vi "Motors sequence 2.vi"(0 "LINX Resource":T1, 1 "Current State":refnum<vi>, 3 "Pole move(microS)":u16(slide) scale=1000.0..2000.0, 4 "Speed(Steps/s)":u32, 5 "Error In":errorcluster, 7 "Wheel":bool, 8 "Spin time/Rest(1)":u32, 9 "Spin n loops":u32=1, 12 "Spin time(2)":u32, 13 "Speed(Steps/s) 2":u32, 14 "Direction":enum16{"CLW", "CCLW", "Off"}(ring), 16 "Pole ms to wait off":u32, 19 "Direction 2":enum16{"CLW", "CCLW", "Off"}(ring), 21 "Seq. iteration 2":refnum<vi>, 22 "Stop":refnum<vi>, 23 "Speed plot 2":refnum<vi>, 24 "Seq. loop":i32, 26 "Spin iteration 2":refnum<vi>) -> (25 "Seq. iteration":i32, 27 "error out":errorcluster)   [LabVIEW 2020]
uses:
  <vilib>/MakerHub/LINX/Private/Type Defs/LINX Ref.ctl
  <vilib>/MakerHub/LINX/Private/Type Defs/Platform.ctl
  <vilib>/MakerHub/LINX/Private/Type Defs/Interface.ctl
  <vilib>/MakerHub/LINX/Private/Device/Type Defs/LINX Device Config.ctl
  <vilib>/MakerHub/LINX/Private/Device/Type Defs/TCP Config.ctl
  <vilib>/MakerHub/LINX/Private/Device/Type Defs/Channels.ctl
  <vilib>/MakerHub/LINX/Public/Sensors/Motion/Servo/Servo Set Pulse Width One Channel.vi
  <vilib>/MakerHub/LINX/Public/Sensors/Motion/Servo/Servo.lvlib
  <vilib>/MakerHub/LINX/LMH-LINX.lvlib
  <vilib>/MakerHub/LINX/Private/Device/Device.lvlib
panel:
  out "Suggested P2 time":u32
  out "Speed plot":dbl(graph)
  out "Spin iteration":i32
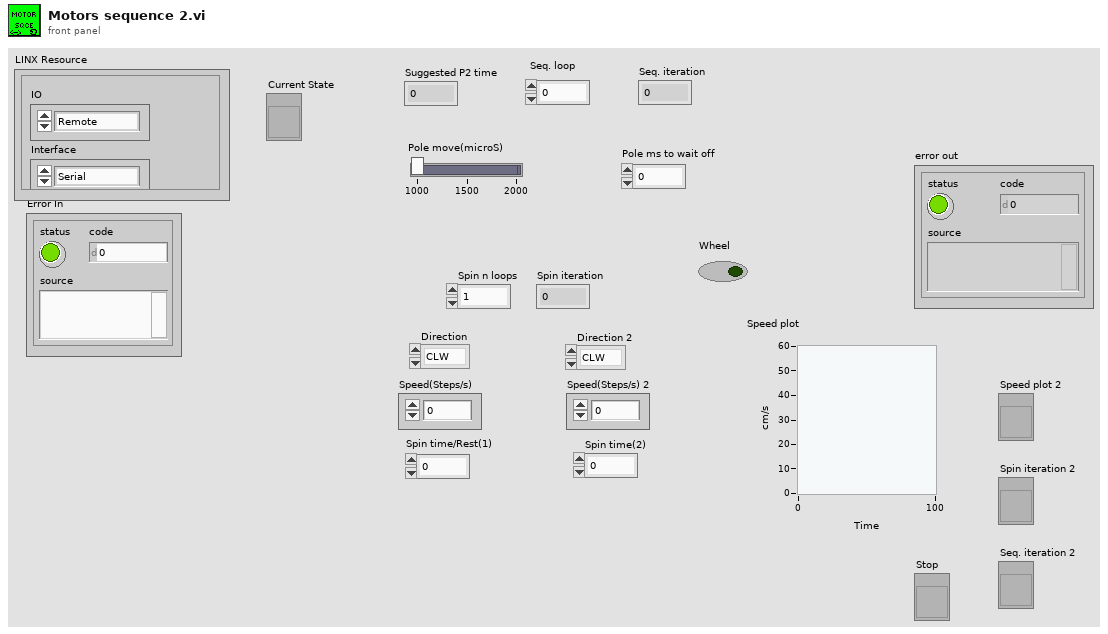
[diagram p1: front panel]
types:
  T1 = typedef "LMH-LINX.lvlib/LINX Ref.ctl" = cluster{"IO":T2, "Interface":T3, "LINX Device Config":T4}
  T2 = typedef "LMH-LINX.lvlib/Platform.ctl" = enum16{"Remote", "Local"}
  T3 = typedef "LMH-LINX.lvlib/Interface.ctl" = enum16{"Serial", "TCP"}
  T4 = typedef "LMH-LINX.lvlib/Device.lvlib/LINX Device Config.ctl" = cluster{"Interface":T3, "COM Port":refnum<visa-resource-name>, "TCP Configuration":T5, "Device Family":u8, "Device ID":u8, "Device Name":string, "TCP Ref":refnum<k5>, "Channels":T6}
  T5 = typedef "LMH-LINX.lvlib/Device.lvlib/TCP Config.ctl" = cluster{"IP Address":string, "Port":u16}
  T6 = typedef "LMH-LINX.lvlib/Channels.ctl" = cluster{"DI":u8[], "DO":u8[], "AI":u8[], "AO":u8[], "PWM":u8[], "QE":u8[], "UART":u8[], "I2C 2":u8[], "SPI":u8[], "CAN":u8[], "Servo":u8[], "AI Ref (V)":dbl, "AI Resolution (Bits)":u8, "AO Ref (V)":dbl, "AO Resolution (Bits)":u8}
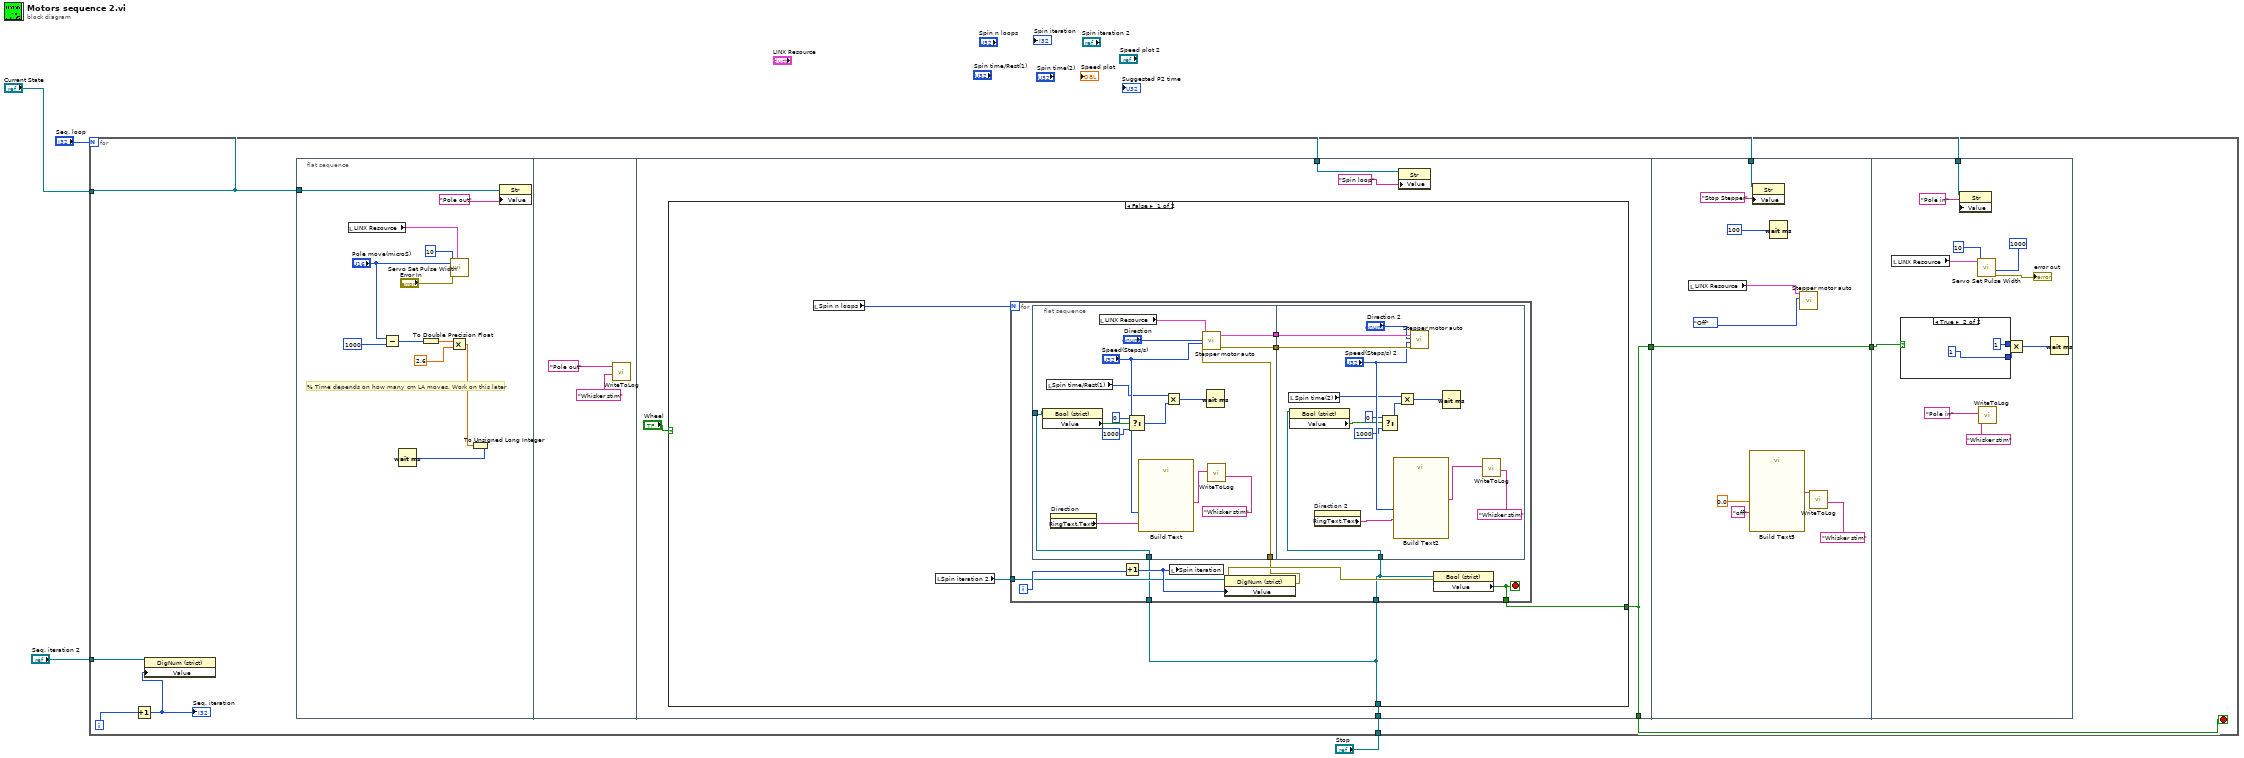
[diagram p0: block diagram]
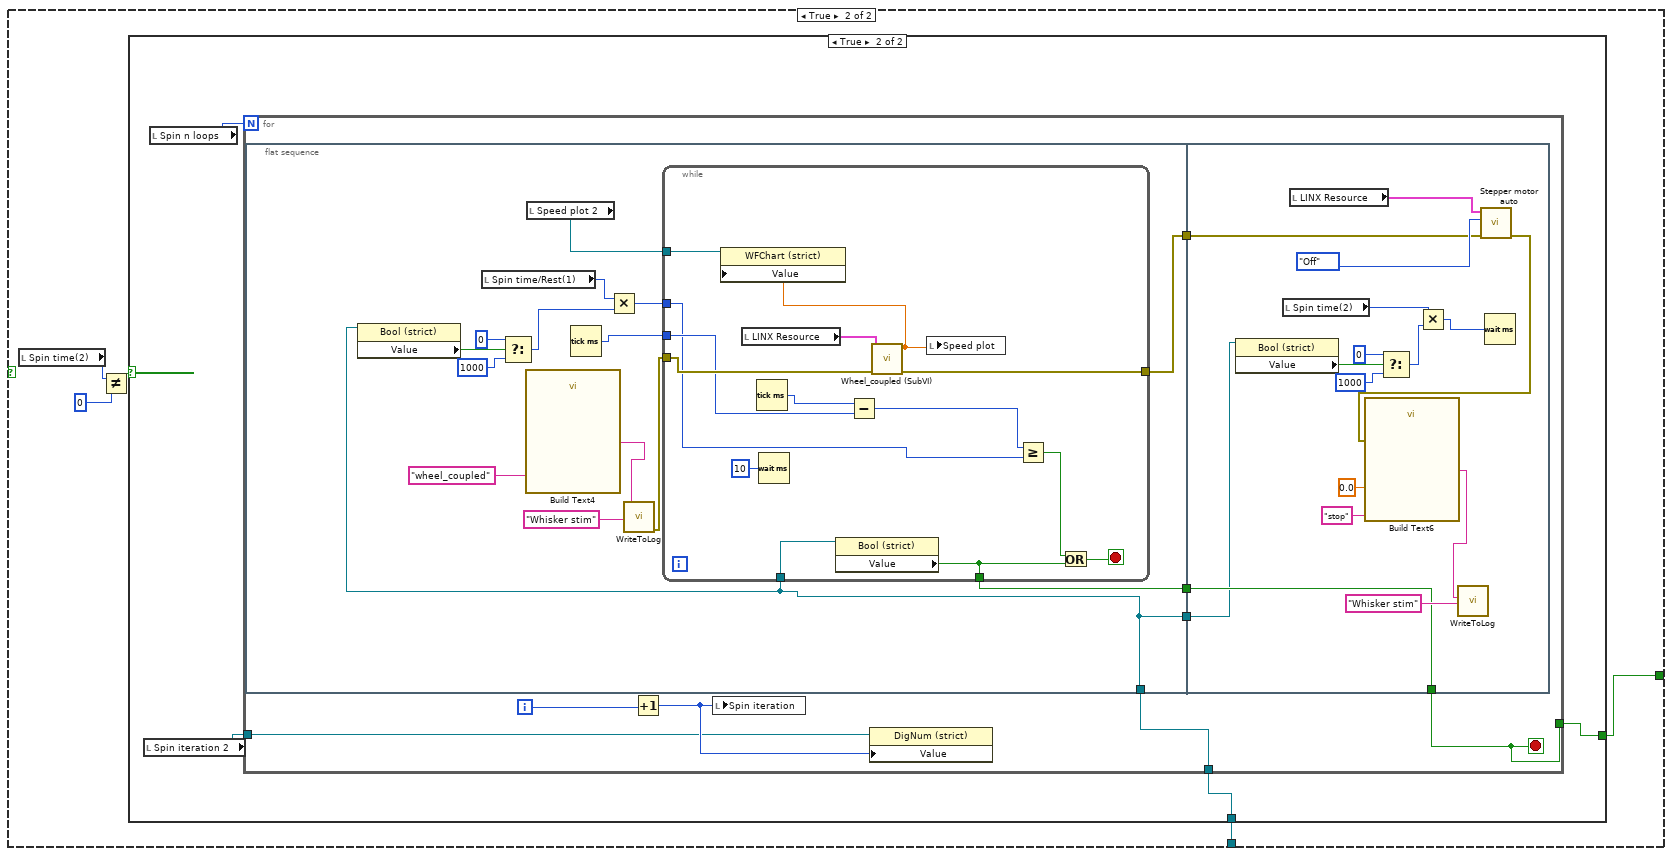
[diagram p2: hidden frame]
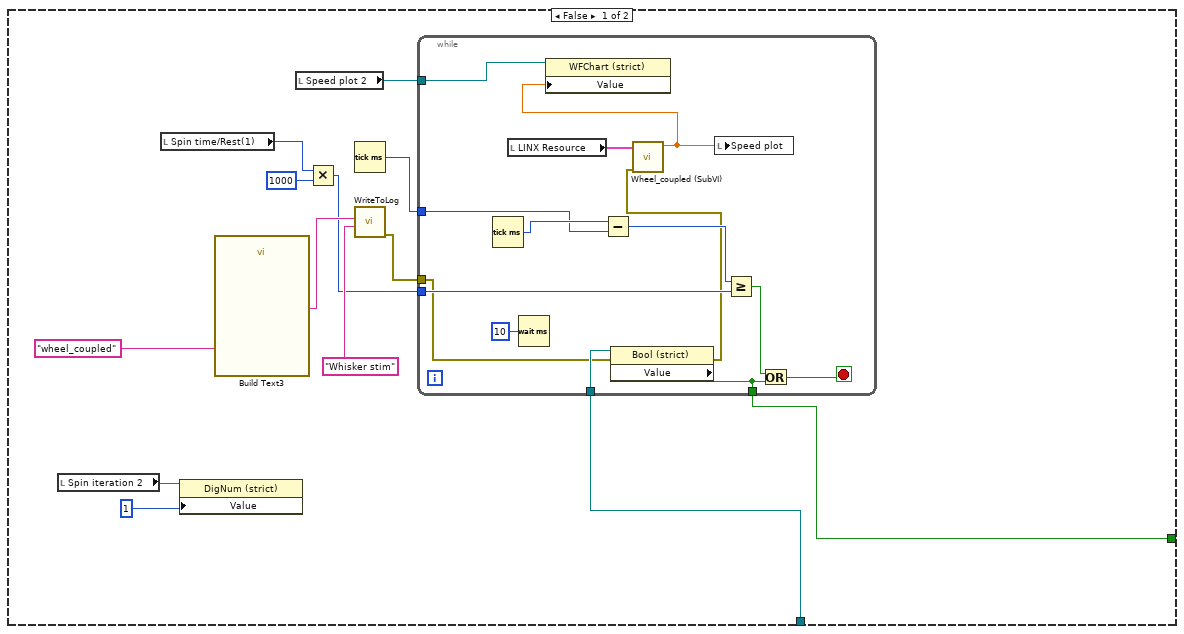
[diagram p3: hidden frame]
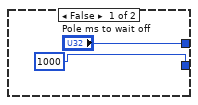
[diagram p4: hidden frame]
diagram:
  n1 = for {
    N: "Seq. loop" -> [_]
    tunnel: "Current State" -> [w12]
    tunnel: "Seq. iteration 2" -> [w9]
    tunnel: "Stop" -> [w8]
    i -> [w11]
    stop <- w7 stop-if-true
    n2 = Increment(x=w11) -> (x+1=w10:i32)
    "Seq. iteration" <- w10
    n3 = property class="DigNum (strict)"(reference=w9, "Value"=w10) -> ()  [unwired: 1 in, 2 out]
    n4 = flat-sequence {
      tunnel: w12 -> [w21]
      tunnel: w12 -> [w29]
      tunnel: w8 -> [w28]
      tunnel: [w27] -> w7
      tunnel: [w27] -> w5
      tunnel: w12 -> [w172]
      tunnel: [w165] -> w6
      tunnel: w5 -> [w165]
      tunnel: w12 -> [w183]
      tunnel: w6 -> [w178]
      frame #0 {
        # "% Time depends on how many cm LA moves. Work on this later"
        n5 = local read "LINX Resource"() -> (w22:T1)
        n6 = Subtract(x="Pole move(microS)", y=u16 1000) -> (x-y=w14:u16)
        n7 = To Double Precision Float(number=w14) -> (double precision float=w13:dbl)
        n8 = call-poly <vilib>:"Servo Set Pulse Width.vi"("Error In"="Error In", "Pulse Width (uS)"="Pole move(microS)", "Servo Channel"=u8 10, "LINX Resource"=w22) -> ()  [unwired: 6 in, 2 out]
        n9 = Multiply(x=w13, y=2.6) -> (x*y=w16:dbl)
        n10 = To Unsigned Long Integer(number=w16) -> (unsigned 32bit integer=w15:u32)
        n11 = Wait (ms)(milliseconds to wait=w15) -> ()  [unwired: 1 out]
        n12 = property class="Str"(reference=w21, "Value"="Pole out" ("State name 2")) -> ()  [unwired: 1 in, 2 out]
      }
      frame #1 {
        n13 = call "WriteToLog.vi"("Category"="Whisker stim", "Message"="Pole out" ("step")) -> ()  [unwired: 9 in, 1 out]
      }
      frame #2 {
        n14 = case shown="False" "Wheel" {
          tunnel: w28 -> [w32 w77]
          tunnel: [w33 w76] -> w27
          frame False {
            n15 = local read "Spin n loops"() -> (w35:u32)
            n16 = local read "Spin iteration 2"() -> (w34:refnum<vi>)
            n17 = for {
              N: w35 -> [_]
              tunnel: w34 -> [w41]
              tunnel: w32 -> [w37]
              tunnel: [w40] -> w33
              tunnel: w32 -> [w36]
              i -> [w42]
              stop <- w40 stop-if-true
              n18 = flat-sequence {
                tunnel: [w58] -> w45
                tunnel: [w57] -> w44
                tunnel: w38 -> [w51]
                tunnel: [w46] -> _
                tunnel: w36 -> [w46]
                tunnel: w45 -> [w73]
                tunnel: w44 -> [w72]
                tunnel: w37 -> [w63]
                frame #0 {
                  n19 = property class="Bool (strict)"(reference=w46) -> ("Value"=w50:bool)  [unwired: 1 in, 2 out]
                  n20 = local read "Spin time/Rest(1)"() -> (w52:u32)
                  n21 = property on="Direction" class="Enum (strict)"() -> ("RingText.Text"=w54:string)  [unwired: 2 in, 2 out]
                  n22 = local read "LINX Resource"() -> (w59:T1)
                  n23 = Select(t=u32 0, s=w50, f=u32 1000 ("y")) -> (s? t:f=w47:u32)
                  n24 = call "Build Text"("speed"="Speed(Steps/s)", "spinmode"=w54) -> ("Result"=w55:string)  [unwired: 12 in, 1 out]
                  n25 = Multiply(x=w52, y=w47) -> (x*y=w61:u32)
                  n26 = call "Stepper motor auto.vi"("Error In"=w51, "Speed(Steps/s)"="Speed(Steps/s)", "Direction"="Direction", "LINX Resource"=w59) -> ("Error Out"=w57:errorcluster, "LINX Resource 2"=w58:T1)  [unwired: 6 in]
                  n27 = Wait (ms)(milliseconds to wait=w61) -> ()  [unwired: 1 out]
                  n28 = call "WriteToLog.vi"("Category"="Whisker stim", "Message"=w55) -> ()  [unwired: 9 in, 1 out]
                }
                frame #1 {
                  n29 = local read "Spin time(2)"() -> (w67:u32)
                  n30 = property class="Bool (strict)"(reference=w63) -> ("Value"=w65:bool)  [unwired: 1 in, 2 out]
                  n31 = property on="Direction 2" class="Enum (strict)"() -> ("RingText.Text"=w69:string)  [unwired: 2 in, 2 out]
                  n32 = Select(t=u32 0, s=w65, f=u32 1000 ("y")) -> (s? t:f=w64:u32)
                  n33 = call "Build Text2"("speed"="Speed(Steps/s) 2", "spinmode"=w69) -> ("Result"=w70:string)  [unwired: 12 in, 1 out]
                  n34 = Multiply(x=w67, y=w64) -> (x*y=w75:u32)
                  n35 = call "Stepper motor auto.vi"("Error In"=w72, "Speed(Steps/s)"="Speed(Steps/s) 2", "Direction"="Direction 2", "LINX Resource"=w73) -> ()  [unwired: 6 in, 2 out]
                  n36 = Wait (ms)(milliseconds to wait=w75) -> ()  [unwired: 1 out]
                  n37 = call "WriteToLog.vi"("Category"="Whisker stim", "Message"=w70) -> ()  [unwired: 9 in, 1 out]
                }
              }
              n38 = Increment(x=w42) -> (x+1=w43:i32)
              n39 = local write "Spin iteration"(w43) -> ()
              n40 = property class="Bool (strict)"(reference=w37) -> (error out=w39:errorcluster, "Value"=w40:bool)  [unwired: 1 in, 1 out]
              n41 = property class="DigNum (strict)"(reference=w41, error in=w39, "Value"=w43) -> (error out=w38:errorcluster)  [unwired: 1 out]
            }
          }
          frame True {
            n42 = local read "Spin time(2)"() -> (w78:u32)
            n43 = Not Equal?(x=w78, y=u32 0) -> (x != y?=w79:bool)
            n44 = case shown="True" w79 {
              tunnel: w77 -> [w87 w109]
              tunnel: [w85 w108] -> w76
              frame False {
                n45 = local read "Spin iteration 2"() -> (w89:refnum<vi>)
                n46 = local read "Spin time/Rest(1)"() -> (w84:u32)
                n47 = property class="DigNum (strict)"(reference=w89, "Value"=1 ("Spin iteration")) -> ()  [unwired: 1 in, 2 out]
                n48 = call "Build Text3"("spinmode"="wheel_coupled" ("Message")) -> ("Result"=w91:string)  [unwired: 13 in, 1 out]
                n49 = local read "Speed plot 2"() -> (w90:refnum<vi>)
                n50 = Multiply(x=w84, y=u32 1000) -> (x*y=w81:u32)
                n51 = Tick Count (ms)() -> (millisecond timer value=w82:u32)
                n52 = call "WriteToLog.vi"("Category"="Whisker stim", "Message"=w91) -> ("error out"=w86:errorcluster)  [unwired: 9 in]
                n53 = while {
                  tunnel: w86 -> [w95]
                  tunnel: w90 -> [w105]
                  tunnel: w87 -> [w103]
                  tunnel: [w101] -> w85
                  tunnel: w82 -> [w96]
                  tunnel: w81 -> [w98]
                  stop <- w102 stop-if-true
                  n54 = Tick Count (ms)() -> (millisecond timer value=w97:u32)
                  n55 = local read "LINX Resource"() -> (w107:T1)
                  n56 = Wait (ms)(milliseconds to wait=u32 10) -> ()  [unwired: 1 out]
                  n57 = Subtract(x=w97, y=w96) -> (x-y=w99:u32)
                  n58 = property class="Bool (strict)"(reference=w103, error in=w95) -> (error out=w94:errorcluster, "Value"=w101:bool)  [unwired: 1 out]
                  n59 = call "Wheel_coupled (SubVI).vi"("Error In"=w94, "LINX Resource"=w107) -> ("Speed plot"=w104:dbl)  [unwired: 8 in, 1 out]
                  n60 = property class="WFChart (strict)"(reference=w105, "Value"=w104) -> ()  [unwired: 1 in, 2 out]
                  n61 = local write "Speed plot"(w104) -> ()
                  n62 = Greater Or Equal?(x=w99, y=w98) -> (x >= y?=w100:bool)
                  n63 = Or(x=w100, y=w101) -> (x .or. y?=w102:bool)
                }
              }
              frame True {
                n64 = local read "Spin iteration 2"() -> (w110:refnum<vi>)
                n65 = local read "Spin n loops"() -> (w111:u32)
                n66 = for {
                  N: w111 -> [_]
                  tunnel: w110 -> [w116]
                  tunnel: w109 -> [w115]
                  tunnel: [w113] -> w108
                  i -> [w118]
                  stop <- w113 stop-if-true
                  n67 = flat-sequence {
                    tunnel: [w131] -> w119
                    tunnel: w115 -> [w120]
                    tunnel: [w128] -> w114
                    tunnel: [w120] -> w112
                    tunnel: w119 -> [w156]
                    tunnel: [w154] -> w113
                    tunnel: w114 -> [w154]
                    tunnel: w112 -> [w149]
                    frame #0 {
                      n68 = property class="Bool (strict)"(reference=w120) -> ("Value"=w124:bool)  [unwired: 1 in, 2 out]
                      n69 = local read "Spin time/Rest(1)"() -> (w127:u32)
                      n70 = Select(t=u32 0, s=w124, f=u32 1000 ("y")) -> (s? t:f=w122:u32)
                      n71 = call "Build Text4"("spinmode"="wheel_coupled" ("Message")) -> ("Result"=w133:string)  [unwired: 13 in, 1 out]
                      n72 = local read "Speed plot 2"() -> (w130:refnum<vi>)
                      n73 = Tick Count (ms)() -> (millisecond timer value=w126:u32)
                      n74 = Multiply(x=w127, y=w122) -> (x*y=w125:u32)
                      n75 = call "WriteToLog.vi"("Category"="Whisker stim", "Message"=w133) -> ("error out"=w129:errorcluster)  [unwired: 9 in]
                      n76 = while {
                        tunnel: w129 -> [w145]
                        tunnel: [w146] -> w131
                        tunnel: w130 -> [w144]
                        tunnel: w120 -> [w142]
                        tunnel: [w140] -> w128
                        tunnel: w126 -> [w138]
                        tunnel: w125 -> [w136]
                        stop <- w141 stop-if-true
                        n77 = local read "LINX Resource"() -> (w148:T1)
                        n78 = Tick Count (ms)() -> (millisecond timer value=w137:u32)
                        n79 = Wait (ms)(milliseconds to wait=u32 10) -> ()  [unwired: 1 out]
                        n80 = property class="Bool (strict)"(reference=w142) -> ("Value"=w140:bool)  [unwired: 1 in, 2 out]
                        n81 = Subtract(x=w137, y=w138) -> (x-y=w135:u32)
                        n82 = call "Wheel_coupled (SubVI).vi"("Error In"=w145, "LINX Resource"=w148) -> ("error out"=w146:errorcluster, "Speed plot"=w143:dbl)  [unwired: 8 in]
                        n83 = property class="WFChart (strict)"(reference=w144, "Value"=w143) -> ()  [unwired: 1 in, 2 out]
                        n84 = local write "Speed plot"(w143) -> ()
                        n85 = Greater Or Equal?(x=w135, y=w136) -> (x >= y?=w139:bool)
                        n86 = Or(x=w139, y=w140) -> (x .or. y?=w141:bool)
                      }
                    }
                    frame #1 {
                      n87 = property class="Bool (strict)"(reference=w149) -> ("Value"=w151:bool)  [unwired: 1 in, 2 out]
                      n88 = local read "Spin time(2)"() -> (w163:u32)
                      n89 = local read "LINX Resource"() -> (w157:T1)
                      n90 = Select(t=u32 0, s=w151, f=u32 1000 ("y")) -> (s? t:f=w150:u32)
                      n91 = Multiply(x=w163, y=w150) -> (x*y=w164:u32)
                      n92 = call "Stepper motor auto.vi"("Error In"=w156, "Direction"=enum16{"CLW", "CCLW", "Off"}."Off", "LINX Resource"=w157) -> ("Error Out"=w155:errorcluster)  [unwired: 7 in, 1 out]
                      n93 = call "Build Text6"("speed"=0.0, "spinmode"="stop" ("Message"), "error in (no error)"=w155) -> ("Result"=w161:string)  [unwired: 11 in, 1 out]
                      n94 = call "WriteToLog.vi"("Category"="Whisker stim", "Message"=w161) -> ()  [unwired: 9 in, 1 out]
                      n95 = Wait (ms)(milliseconds to wait=w164) -> ()  [unwired: 1 out]
                    }
                  }
                  n96 = Increment(x=w118) -> (x+1=w117:i32)
                  n97 = local write "Spin iteration"(w117) -> ()
                  n98 = property class="DigNum (strict)"(reference=w116, "Value"=w117) -> ()  [unwired: 1 in, 2 out]
                }
              }
            }
          }
        }
        n99 = property class="Str"(reference=w29, "Value"="Spin loop" ("State name")) -> ()  [unwired: 1 in, 2 out]
      }
      frame #3 {
        n100 = local read "LINX Resource"() -> (w169:T1)
        n101 = call "Build Text5"("speed"=0.0, "spinmode"="off") -> ("Result"=w171:string)  [unwired: 12 in, 1 out]
        n102 = property class="Str"(reference=w172, "Value"="Stop Stepper" ("State name")) -> ()  [unwired: 1 in, 2 out]
        n103 = Wait (ms)(milliseconds to wait=u32 100) -> ()  [unwired: 1 out]
        n104 = call "Stepper motor auto.vi"("Direction"=enum16{"CLW", "CCLW", "Off"}."Off", "LINX Resource"=w169) -> ()  [unwired: 8 in, 2 out]
        n105 = call "WriteToLog.vi"("Category"="Whisker stim", "Message"=w171) -> ()  [unwired: 9 in, 1 out]
      }
      frame #4 {
        n106 = local read "LINX Resource"() -> (w179:T1)
        n107 = case shown="True" w178 {
          tunnel: [u32 1000 ("y") u32 1 ("y")] -> w176
          tunnel: ["Pole ms to wait off" u32 1 ("Pole ms to wait off")] -> w175
          frame False {
          }
          frame True {
          }
        }
        n108 = property class="Str"(reference=w183, "Value"="Pole in" ("State name")) -> ()  [unwired: 1 in, 2 out]
        n109 = call-poly <vilib>:"Servo Set Pulse Width.vi"("Pulse Width (uS)"=u16 1000, "Servo Channel"=u8 10, "LINX Resource"=w179) -> ("Error Out"=→"error out":errorcluster)  [unwired: 7 in, 1 out]
        n110 = call "WriteToLog.vi"("Category"="Whisker stim", "Message"="Pole in" ("step")) -> ()  [unwired: 9 in, 1 out]
        n111 = Multiply(x=w175, y=w176) -> (x*y=w177:u32)
        n112 = Wait (ms)(milliseconds to wait=w177) -> ()  [unwired: 1 out]
      }
    }
  }
